vi "Save Report.vi"(8 "error in":errorcluster, 9 "Array - Dots":dbl[][](array[numeric]), 10 "Temp array":dbl[](array[numeric]), 11 "Исходные данные":T1) -> (0 "error out":errorcluster)   [LabVIEW 2023, in "AutoPV.lvlib"]
uses:
  AutoPV.lvlib
  Initial Data/InitalData Type.ctl
  <vilib>/Utility/sysdir.llb/System Directory Type.ctl
  <vilib>/Utility/file.llb/Write Delimited Spreadsheet (string).vi
  Initial Data/Initial Data.lvlib
panel:
  out "Array":string[][](array[string])
  out "Array of Headers":string[](array[string])
  out "Array of Data":string[](array[string])
  # "Образец"
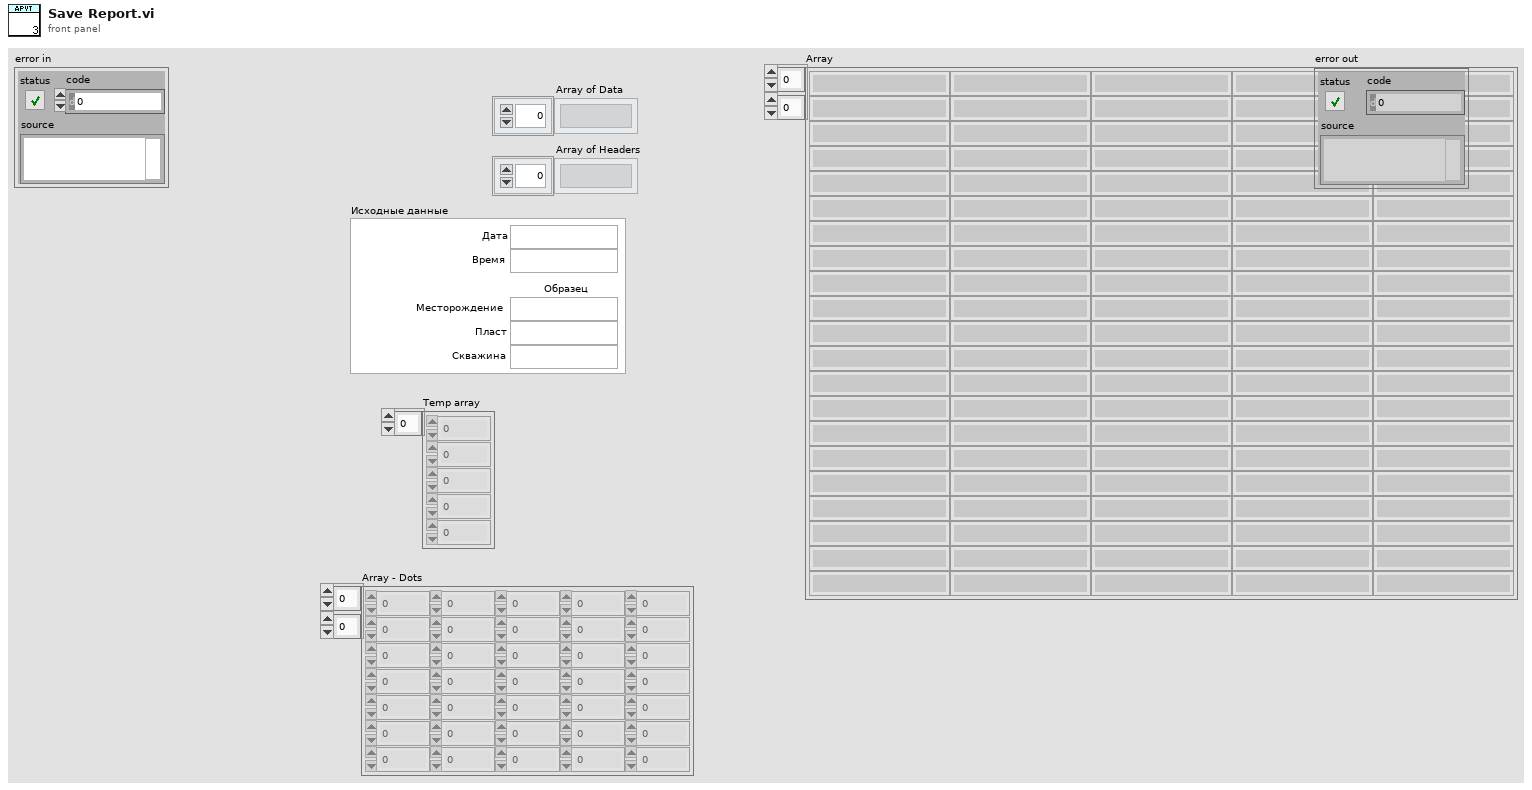
[diagram p1: front panel]
types:
  T1 = typedef "Initial Data.lvlib/InitalData Type.ctl" = cluster{"Дата":string, "Время":string, "Месторождение":string, "Пласт":string, "Скважина":string}
  T2 = typedef "System Directory Type.ctl" = i32
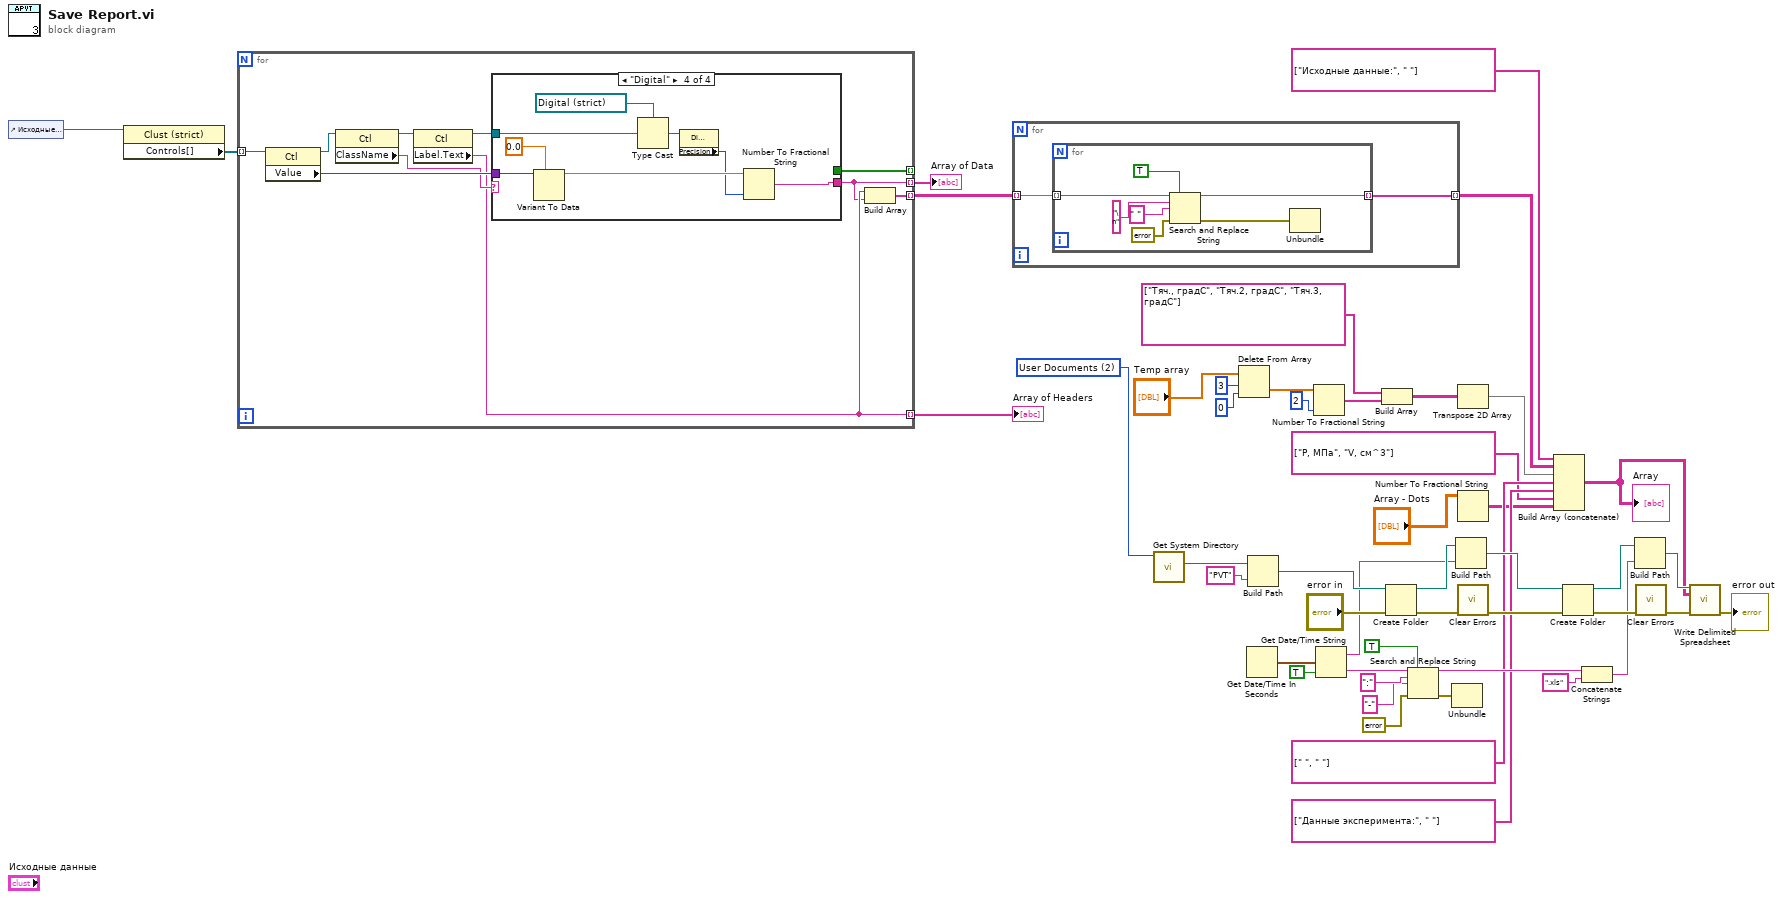
[diagram p0: block diagram]
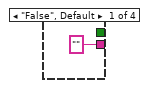
[diagram p2: hidden frame]
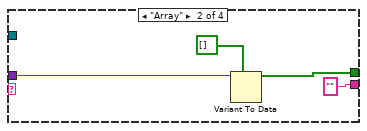
[diagram p3: hidden frame]
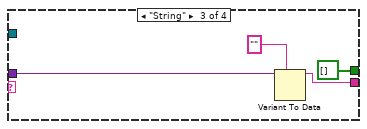
[diagram p4: hidden frame]
diagram:
  w44 = T2 2 items=["User Home"=0, "User Desktop"=1, "User Documents"=2, "User Application Data"=3, "User Preferences"=4, "User Temporary"=5, "Public Documents"=6, "Public Application Data"=7, "Public Preferences"=8, "Public Cache"=13, "System Core Libraries"=9, "System Installed Libraries"=10, "Application Files"=11, "Boot Volume Root"=12] ("system directory type")
  n1 = control-ref of="Исходные данные"() -> (w46:refnum<vi>)
  n2 = property class="Clust (strict)"(reference=w46) -> ("Controls[]"=w48:refnum<vi>[])  [unwired: 1 in, 2 out]
  n3 = for {
    tunnel: w48 -> [w58] mode=indexing
    tunnel: [w50] -> w47 mode=indexing
    tunnel: [w51] -> w45 mode=indexing
    tunnel: [w54] -> _ mode=indexing
    tunnel: [w49] -> w29 mode=indexing
    n4 = property class="Ctl"(reference=w58) -> (reference out=w56:refnum<vi>, "Value"=w57:variant)  [unwired: 1 in, 1 out]
    n5 = property class="Ctl"(reference=w56) -> (reference out=w55:refnum<vi>, "ClassName"=w53:string)  [unwired: 1 in, 1 out]
    n6 = property class="Ctl"(reference=w55) -> (reference out=w52:refnum<vi>, "Label.Text"=w51:string)  [unwired: 1 in, 1 out]
    n7 = case shown="\"Digital\"" w53 {
      tunnel: w57 -> [_ w62 w66 w75]
      tunnel: ["" "" w65 w72] -> w50
      tunnel: [_ w61 bool[] [] ("Array 2") _] -> w54
      tunnel: w52 -> [_ _ _ w71]
      frame "False", Default {
      }
      frame "Array" {
        n8 = Variant To Data(type=bool[] [] ("Array 2"), Variant=w62) -> (data=w61:bool[])  [unwired: 1 in, 1 out]
      }
      frame "String" {
        n9 = Variant To Data(type="", Variant=w66) -> (data=w65:string)  [unwired: 1 in, 1 out]
      }
      frame "Digital" {
        n10 = Variant To Data(type=0.0, Variant=w75) -> (data=w73:dbl)  [unwired: 1 in, 1 out]
        n11 = Type Cast(type=refnum<vi> refnum ("Numeric"), x=w71) -> (*(type *) &x=w69:refnum<vi>)
        n12 = property class="DigNum (strict)"(reference=w69) -> ("Precision"=w68:u8)  [unwired: 1 in, 2 out]
        n13 = Number To Fractional String(number=w73, precision (6)=w68) -> (F-format string=w72:string)  [unwired: 2 in]
      }
    }
    n14 = Build Array(w51, w50) -> (w49:string[])
  }
  "Array of Data" <- w47
  "Array of Headers" <- w45
  n15 = for {
    tunnel: w29 -> [w77] mode=indexing
    tunnel: [w76] -> w28 mode=indexing
    n16 = for {
      tunnel: w77 -> [w84] mode=indexing
      tunnel: [w81] -> w76 mode=indexing
      n17 = Search and Replace String(replace all?=TRUE ("replace all? (F)"), input string=w84, search string="\n", replace string=" " ("replace string (\"\")"), error in=errorcluster {"status"=FALSE, "code"=0, "source"=""} ("error in (no error)")) -> (result string=w81:string, error out=w82:errorcluster)  [unwired: 3 in, 2 out]
      n18 = Unbundle(w82) -> ()  [unwired: 3 out]
    }
  }
  n19 = call <vilib>:"Get System Directory.vi"("system directory type"=w44) -> ("system directory"=w43:path)  [unwired: 10 in]
  n20 = Delete From Array(array="Temp array", length=3, index=0) -> (deleted portion=w1:dbl[])  [unwired: 1 out]
  n21 = Get Date/Time In Seconds() -> (seconds since 1Jan1904=w35:timestamp)
  n22 = Build Path(base path=w43, name or relative path="PVT") -> (appended path=w40:path)
  n23 = Number To Fractional String(number=w1, precision (6)=i16 2) -> (F-format string=w15:string[])  [unwired: 2 in]
  n24 = Get Date/Time String(seconds (now)=w35, want seconds? (F)=TRUE) -> (date string=w33:string, time string=w19:string)  [unwired: 1 in]
  n25 = Build Array(string[] ["Тяч., градС", "Тяч.2, градС", "Тяч.3, градС"], w15) -> (w14:string[][])
  n26 = Create Folder(path (use dialog)=w40, error in="error in") -> (created path=w36:path, error out=w41:errorcluster)  [unwired: 1 in, 1 out]
  n27 = Search and Replace String(replace all?=TRUE ("replace all? (F)"), input string=w19, search string=":", replace string="-" ("replace string (\"\")"), error in=errorcluster {"status"=FALSE, "code"=0, "source"=""} ("error in (no error)")) -> (result string=w18:string, error out=w23:errorcluster)  [unwired: 3 in, 2 out]
  n28 = Unbundle(w23) -> ()  [unwired: 3 out]
  n29 = Build Path(base path=w36, name or relative path=w33) -> (appended path=w32:path)
  n30 = Transpose 2D Array(2D array=w14) -> (transposed array=w12:string[][])
  n31 = Number To Fractional String(number="Array - Dots") -> (F-format string=w5:string[][])  [unwired: 3 in]
  n32 = call <vilib>:"Clear Errors.vi"("error in (no error)"=w41) -> ("error out"=w38:errorcluster)  [unwired: 5 in, 1 out]
  n33 = Build Array (concatenate)(string[] ["Исходные данные:", " "], w28, w12, string[] [" ", " "], string[] ["Данные эксперимента:", " "], string[] ["Р, МПа", "V, см^3"], w5) -> (w13:string[][])
  "Array" <- w13
  n34 = Create Folder(path (use dialog)=w32, error in=w38) -> (created path=w31:path, error out=w37:errorcluster)  [unwired: 1 in, 1 out]
  n35 = Concatenate Strings(w18, ".xls" ("string")) -> (w26:string)
  n36 = Build Path(base path=w31, name or relative path=w26) -> (appended path=w30:path)
  n37 = call <vilib>:"Clear Errors.vi"("error in (no error)"=w37) -> ("error out"=w27:errorcluster)  [unwired: 5 in, 1 out]
  n38 = call-poly <vilib>:"Write Delimited Spreadsheet.vi"("file path (dialog if empty)"=w30, "2D data"=w13, "error in (no error)"=w27) -> ("error out"=→"error out":errorcluster)  [unwired: 11 in, 1 out]
